vi "Get Single Value from Double Array.vi"(11 "values":dbl[](array[numeric])) -> (2 "multiple values":bool, 3 "single value":dbl)   [LabVIEW 2017, in "NI_Robotics_Configure Steering Frame.lvlib" / "User Defined Frame Subpanel.lvlib"]
uses:
  <vilib>/robotics/Dialog/Configure Steering Frame/User Defined Frame Subpanel/User Defined Frame Subpanel.lvlib
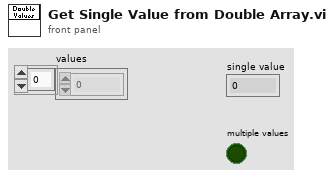
[diagram p1: front panel]
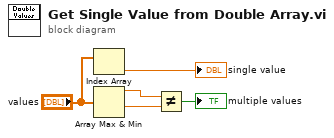
[diagram p0: block diagram]
diagram:
  n1 = Index Array(array="values") -> (element=→"single value":dbl)  [unwired: 1 in]
  n2 = Array Max & Min(array="values") -> (max value=w4:dbl, min value=w5:dbl)  [unwired: 2 out]
  n3 = Not Equal?(x=w4, y=w5) -> (x != y?=→"multiple values":bool)
